vi "Address Space Size.vi"(2 "niInstr AXI4-Lite address space v1 FPGA in":refnum<class "niInstr AXI4-Lite Address Space v1 FPGA.lvclass">) -> (6 "size":u32)   [LabVIEW 2015, in "niInstr AXI4-Lite Address Space v1 FPGA.lvclass"]
doc: "returns the size of the address space.\n\n<B>Input Parameters</B>\n\n<B>niInstr AXI4-Lite address space v1 FPGA in</B> is the AXI4-Lite address space to use.\n\n<B>Output Parameters</B>\n\n<B>size</B> is the size of the address space."
uses:
  <instrlib>/_niInstr/CLIP Adapters/v1/FPGA/AXI4-Lite/Address Space/niInstr AXI4-Lite Address Space v1 FPGA.lvclass
  <instrlib>/_niInstr/CLIP Adapters/v1/FPGA/AXI4-Lite/Address Space/niInstr AXI4-Lite Address Space v1 FPGA.lvclass/niInstr AXI4-Lite Address Space v1 FPGA.ctl
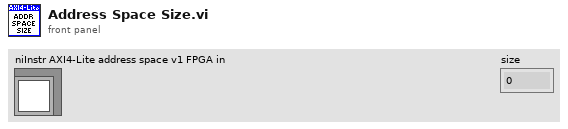
[diagram p1: front panel]
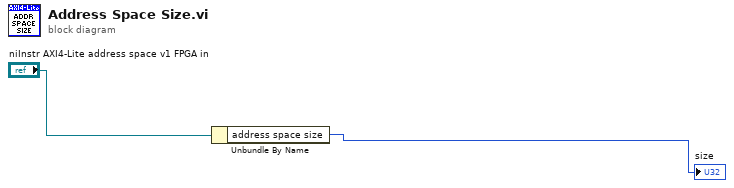
[diagram p0: block diagram]
diagram:
  n1 = Unbundle By Name("niInstr AXI4-Lite address space v1 FPGA in") -> ("address space size"=→"size":u32)
